vi "open.vi"(8 "error in (no error)":errorcluster caption="错误输入（无错误）", 10 "database":string, 11 "access 输入":refnum<class "access.lvclass">) -> (0 "error out":errorcluster caption="错误输出", 3 "access 输出":refnum<class "access.lvclass">)   [LabVIEW 2016, in "中水三立SQL数据传输.lvlib" / "access.lvclass"]
uses:
  access.lvclass
  <vilib>/Utility/sysdir.llb/System Directory Type.ctl
  database_class/database.lvclass/database.ctl
  <vilib>/addons/database/Connection.llb/DB Tools Open Connec (String).vi
  <vilib>/addons/database/NI_Database_API.lvlib
  database_class/database.lvclass
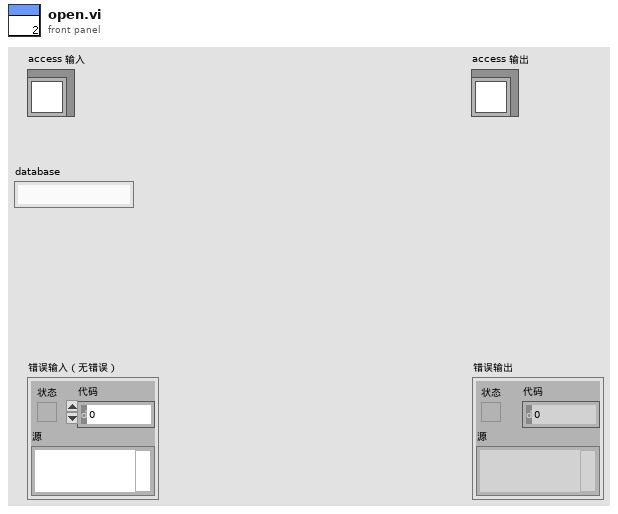
[diagram p1: front panel]
types:
  T1 = typedef "System Directory Type.ctl" = i32
  T2 = typedef "NI_Database_API.lvlib/Conn ObjectReference.ctl" = refnum<k1>
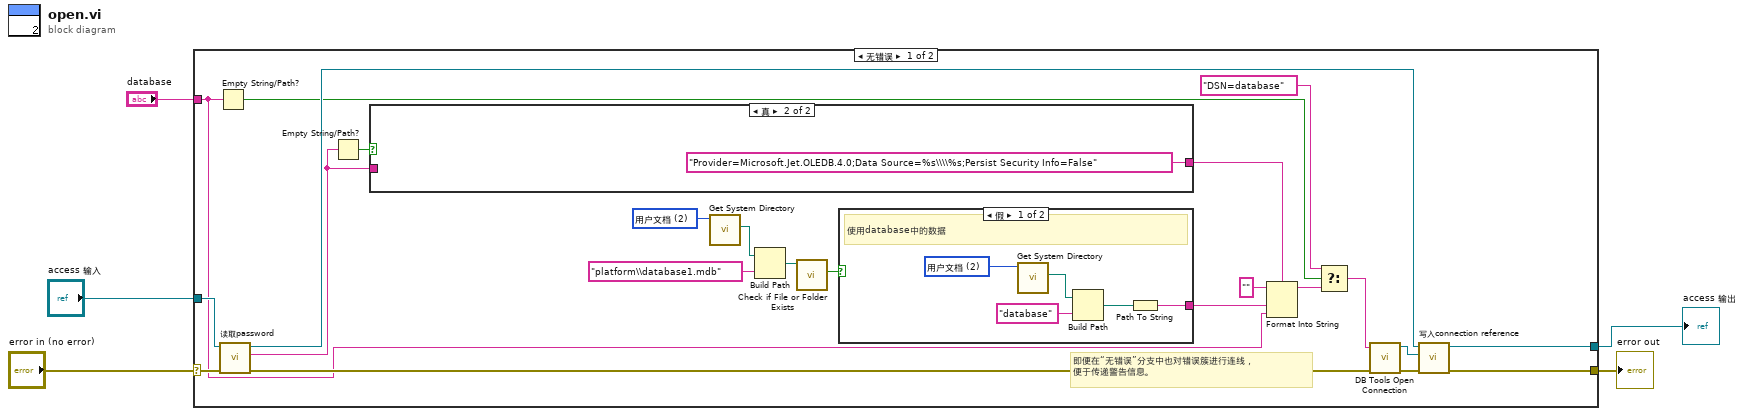
[diagram p0: block diagram]
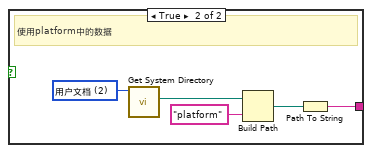
[diagram p2: hidden frame]
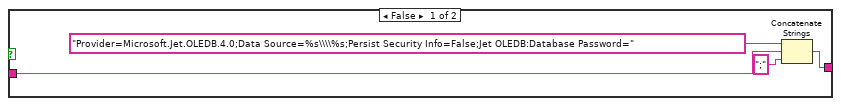
[diagram p3: hidden frame]
diagram:
  n1 = case shown="无错误" "error in (no error)" {
    selector: "error in (no error)" -> [w17 w44]
    tunnel: "access 输入" -> [w19 w45]
    tunnel: [w13 w45] -> w5
    tunnel: "database" -> [w10 _]
    tunnel: [w11 w44] -> w3
    frame No Error {
      w25 = T1 2 items=["用户目录"=0, "用户桌面"=1, "用户文档"=2, "用户应用程序数据"=3, "用户设置"=4, "用户临时目录"=5, "公共文档"=6, "公共应用程序数据"=7, "公共设置"=8, "公共缓存"=13, "系统核心库"=9, "系统安装库"=10, "应用程序文件"=11, "启动盘根目录"=12] ("system directory type")
      # "即便在“无错误”分支中也对错误簇进行连线，\n便于传递警告信息。"
      n2 = Empty String/Path?(string/path=w10) -> (empty?=w9:bool)
      n3 = call "读取password.vi"("error in (no error)"=w17, "database输入"=w19) -> ("error out"=w16:errorcluster, "password"=w18:string, "database输出"=w15:refnum<class "access.lvclass">)  [unwired: 7 in]
      n4 = Empty String/Path?(string/path=w18) -> (empty?=w28:bool)
      n5 = case shown="真" w28 {
        tunnel: [w39 "Provider=Microsoft.Jet.OLEDB.4.0;Data Source=%s\\\\%s;Persist Security Info=False" ("格式字符串")] -> w20
        tunnel: w18 -> [w42 _]
        frame False {
          n6 = Concatenate Strings("Provider=Microsoft.Jet.OLEDB.4.0;Data Source=%s\\\\%s;Persist Security Info=False;Jet OLEDB:Database Password=" ("格式字符串"), w42, ";" ("字符串")) -> (w39:string)
        }
        frame True {
        }
      }
      n7 = call <vilib>:"Get System Directory.vi"("system directory type"=w25) -> ("system directory"=w26:path)  [unwired: 10 in]
      n8 = Build Path(base path=w26, name or relative path="platform\\database1.mdb" ("condition")) -> (appended path=w24:path)
      n9 = call <vilib>:"Check if File or Folder Exists.vi"("path"=w24) -> ("file or folder exists?"=w22:bool)  [unwired: 8 in, 2 out]
      n10 = case shown="假" w22 {
        tunnel: [w29 w34] -> w21
        frame False {
          w32 = T1 2 items=["用户目录"=0, "用户桌面"=1, "用户文档"=2, "用户应用程序数据"=3, "用户设置"=4, "用户临时目录"=5, "公共文档"=6, "公共应用程序数据"=7, "公共设置"=8, "公共缓存"=13, "系统核心库"=9, "系统安装库"=10, "应用程序文件"=11, "启动盘根目录"=12] ("system directory type")
          # "使用database中的数据"
          n11 = call <vilib>:"Get System Directory.vi"("system directory type"=w32) -> ("system directory"=w31:path)  [unwired: 10 in]
          n12 = Build Path(base path=w31, name or relative path="database" ("condition")) -> (appended path=w33:path)
          n13 = Path To String(path=w33) -> (string=w29:string)
        }
        frame True {
          w38 = T1 2 items=["用户目录"=0, "用户桌面"=1, "用户文档"=2, "用户应用程序数据"=3, "用户设置"=4, "用户临时目录"=5, "公共文档"=6, "公共应用程序数据"=7, "公共设置"=8, "公共缓存"=13, "系统核心库"=9, "系统安装库"=10, "应用程序文件"=11, "启动盘根目录"=12] ("system directory type")
          # "使用platform中的数据"
          n14 = call <vilib>:"Get System Directory.vi"("system directory type"=w38) -> ("system directory"=w37:path)  [unwired: 10 in]
          n15 = Build Path(base path=w37, name or relative path="platform" ("condition")) -> (appended path=w35:path)
          n16 = Path To String(path=w35) -> (string=w34:string)
        }
      }
      n17 = Format Into String(format string=w20, initial string="" ("初始字符串"), w21, w10) -> (resulting string=w7:string)  [unwired: 1 in, 1 out]
      n18 = Select(t="DSN=database", s=w9, f=w7) -> (s? t:f=w6:string)
      n19 = call-poly <vilib>:"DB Tools Open Connection.vi"("error in (no error)"=w16, "connection information"=w6) -> ("error out"=w12:errorcluster, "connection reference"=w14:T2)  [unwired: 6 in]
      n20 = call-dynamic "写入connection reference.vi"("error in (no error)"=w12, "reference"=w14, "database输入"=w15) -> ("error out"=w11:errorcluster, "database输出"=w13:refnum<class "access.lvclass">)  [unwired: 7 in]
    }
    frame Error {
    }
  }
  "error out" <- w3
  "access 输出" <- w5
